vi "XML Script - ToXMLString.vi"   [LabVIEW 2020]
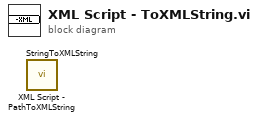
[diagram p0: block diagram]
diagram:
  n1 = call <vilib>:"XML Script - PathToXMLString.vi"() -> ()  [unwired: 1 in, 1 out]
  n2 = call <vilib>:"StringToXMLString.vi"() -> ()  [unwired: 1 in, 1 out]
